vi "stringtohex.vi"(11 "Hash String":string) -> (3 "string":string)   [LabVIEW 2020]
panel:
  out "Array":u8[](array[numeric]) format="%.0x"
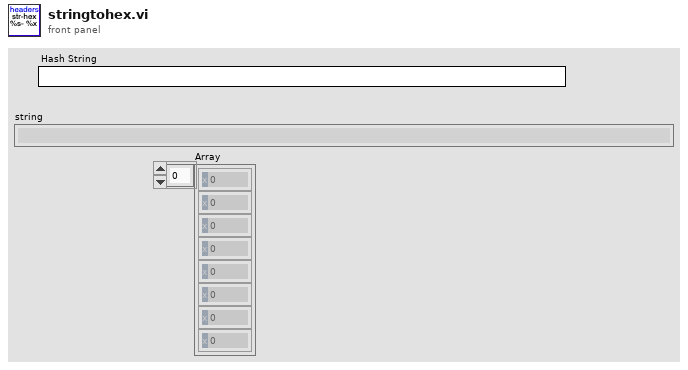
[diagram p1: front panel]
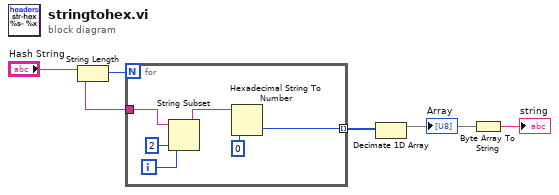
[diagram p0: block diagram]
diagram:
  n1 = String Length(string="Hash String") -> (length=w1:i32)
  n2 = for {
    N: w1 -> [_]
    tunnel: "Hash String" -> [w9]
    tunnel: [w11] -> w4 mode=indexing
    i -> [w8]
    n3 = String Subset(string=w9, offset (0)=w8, length (rest)=2 ("length (rest)")) -> (substring=w6:string)
    n4 = Hexadecimal String To Number(string=w6, default (0uL)=u8 0) -> (number=w11:u8)  [unwired: 1 in, 1 out]
  }
  n5 = Decimate 1D Array(w4) -> (w3:u8[])  [unwired: 1 out]
  "Array" <- w3
  n6 = Byte Array To String(unsigned byte array=w3) -> (string=→"string":string)
